vi "过滤数组元素[U32](冲突时的文件备份2013-03-27 14-09-23).vi"(8 "error in (no error)":errorcluster caption="错误输入（无错误）", 10 "过滤元素":u32[](array[numeric]), 11 "输入数组":u32[](array[numeric])) -> (0 "error out":errorcluster caption="错误输出", 2 "已过滤元素索引":i32[](array[numeric]), 3 "输出数组":u32[](array[numeric]))   [LabVIEW 2012]
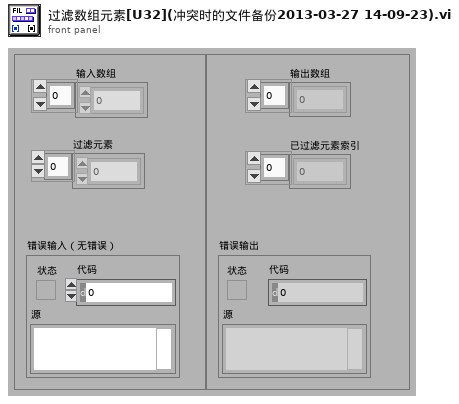
[diagram p1: front panel]
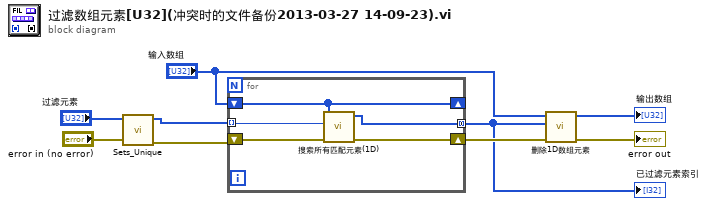
[diagram p0: block diagram]
diagram:
  n1 = call-poly "Sets_Unique.vi"("error in (no error)"="error in (no error)", "输入数组"="过滤元素") -> ("error out"=w3:errorcluster, "输出数组"=w1:u32[])  [unwired: 7 in, 1 out]
  n2 = for {
    tunnel: w1 -> [w12] mode=indexing
    shift-right: [w11] -> _
    shift-left: "输入数组" -> [w11]
    shift-right: [w13] -> w8
    shift-left: w3 -> [w14]
    tunnel: [w10] -> w5 mode=concatenating
    n3 = call-poly "搜索所有匹配元素(1D).vi"("error in (no error)"=w14, "元素"=w12, "数组"=w11) -> ("error out"=w13:errorcluster, "匹配元素索引"=w10:i32[])  [unwired: 6 in, 1 out]
  }
  "已过滤元素索引" <- w5
  n4 = call-poly "删除1D数组元素.vi"("error in (no error)"=w8, "索引"=w5, "输入数组"="输入数组") -> ("error out"=→"error out":errorcluster, "剩余元素"=→"输出数组":u32[])  [unwired: 6 in, 1 out]
